vi "setFPGA.vi"(10 "FPGA":refnum<class "FPGA.lvclass">, 11 "ModbusSubnetBTxDataFIFO in":refnum<class "ModbusSubnetBTxDataFIFO.lvclass">) -> (3 "ModbusSubnetBTxDataFIFO out":refnum<class "ModbusSubnetBTxDataFIFO.lvclass">)   [LabVIEW 2016, in "ModbusSubnetBTxDataFIFO.lvclass"]
uses:
  ModbusSubnetBTxDataFIFO.lvclass
  FPGA/FPGA.lvclass
  ModbusSubnetBTxDataFIFO.lvclass/ModbusSubnetBTxDataFIFO.ctl
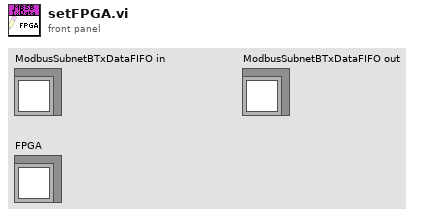
[diagram p1: front panel]
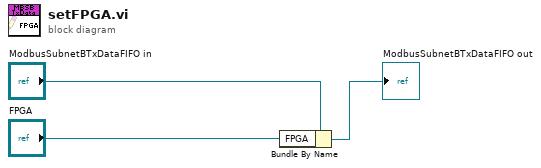
[diagram p0: block diagram]
diagram:
  n1 = Bundle By Name(cluster="ModbusSubnetBTxDataFIFO in", "FPGA"="FPGA") -> (→"ModbusSubnetBTxDataFIFO out":refnum<class "ModbusSubnetBTxDataFIFO.lvclass">)
